vi "CoolLED_Control_v1.0.vi"(8 "error in":errorcluster) -> (0 "error out":errorcluster)   [LabVIEW 2025]
uses:
  SubVIs/States.ctl
  <vilib>/Instr/_visa.llb/VISA Configure Serial Port (Instr).vi
panel:
  in  "Tab Control":enum32{"Commands", "Expert"}(tab)
  in  "Presets":enum16{"DAPI", "GFP", "RFP", "None", "Multiple"}(ring)=enum."None"
  in  "Store":bool
  in  "Cluster":T1 {"Green-Red" step=1 scale=0.0..100.0; "Blue" step=1 scale=0.0..100.0; "Violet" step=1 scale=0.0..100.0}
  in  "VISA resource name":refnum<visa-resource-name>="COM5"
  out "Current command":string="CSSAXF000BXF000CXF000\r\n"
  in  "Stop":bool
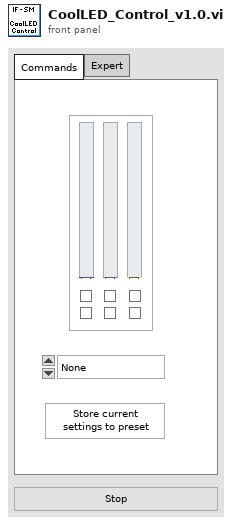
[diagram p1: front panel]
types:
  T1 = cluster{"Violet":u8, "Blue":u8, "Green-Red":u8, "A(S)Selected/(N)Unselected":bool, "B(S)Selected/(N)Unselected":bool, "C(S)Selected/(N)Unselected":bool, "A(N)ON/(F)OFF":bool, "(N)ON/(F)OFF":bool, "C(N)ON/(F)OFF":bool}
  T2 = typedef "States.ctl" = enum16{"Initialize", "Wait for Event", "Close", "Store", "Send", "Create_command", "Presets"}
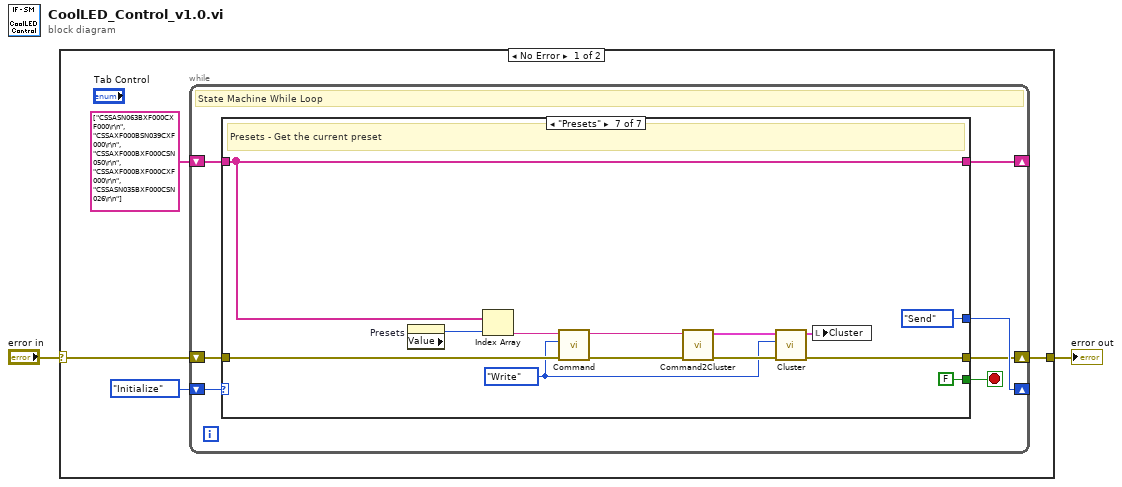
[diagram p0: block diagram]
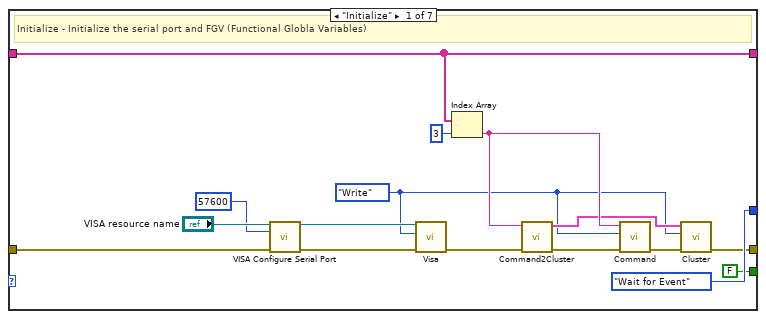
[diagram p2: hidden frame]
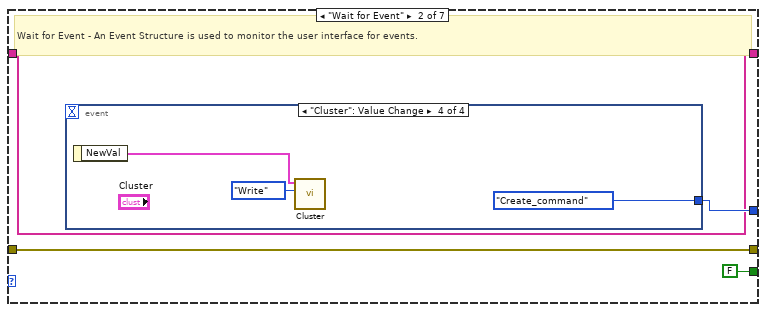
[diagram p3: hidden frame]
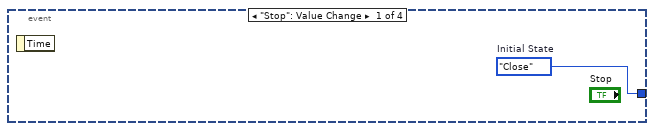
[diagram p4: hidden frame]
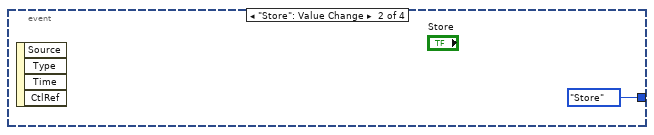
[diagram p5: hidden frame]
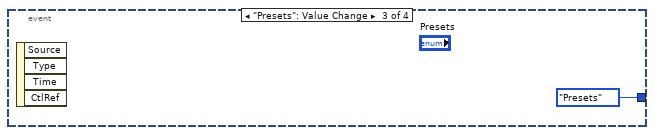
[diagram p6: hidden frame]
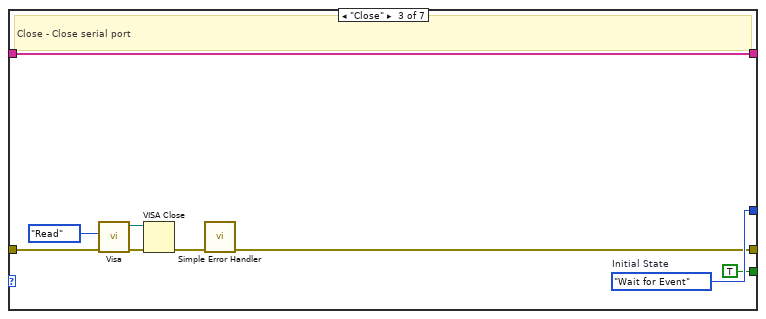
[diagram p7: hidden frame]
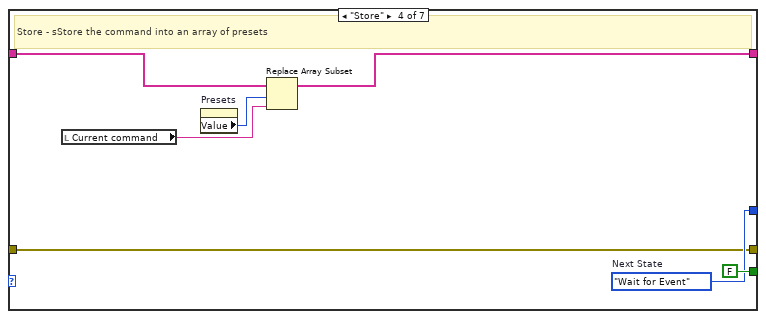
[diagram p8: hidden frame]
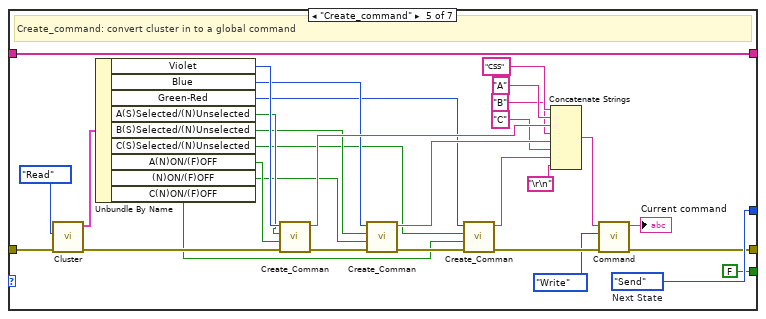
[diagram p9: hidden frame]
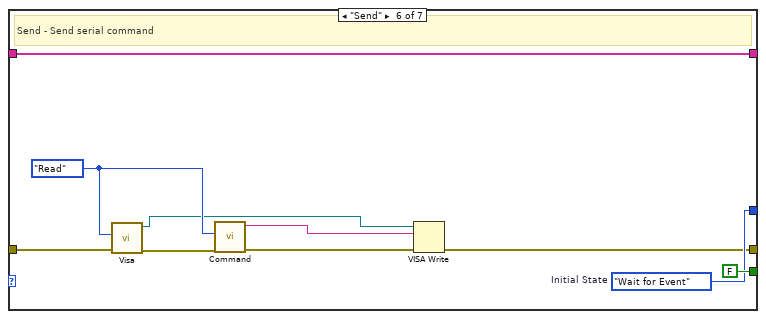
[diagram p10: hidden frame]
diagram:
  n1 = case shown="No Error" "error in" {
    selector: "error in" -> [w5 w110]
    tunnel: [w4 w110] -> w1
    frame No Error {
      n2 = while {
        shift-right: [w13] -> _
        shift-left: States."Initialize" ("Initial State") -> [w11]
        shift-right: [w9] -> w4
        shift-left: w5 -> [w10]
        shift-right: [w7] -> _
        shift-left: string[] ["CSSASN063BXF000CXF000\r\n", "CSSAXF000BSN039CXF000\r\n", "CSSAXF000BXF000CSN050\r\n", "CSSAXF000BXF000CXF000\r\n", "CSSASN035BXF000CSN026\r\n"] ("output array") -> [w8]
        stop <- w12 stop-if-true
        # "State Machine While Loop"
        n3 = case "State Machine Case Structure" shown="\"Presets\"" w11 {
          tunnel: [States."Wait for Event" ("Initial State") w33 w48 w54 w86 w95 States."Send" ("Initial State")] -> w13
          tunnel: [FALSE ("Stop the Loop") FALSE ("Stop the Loop") TRUE ("Stop the Loop") FALSE ("Stop the Loop") FALSE ("Stop the Loop") FALSE ("Stop the Loop") FALSE ("Stop the Loop")] -> w12
          tunnel: w10 -> [w26 w31 w43 w53 w68 w90 w106]
          tunnel: [w16 w31 w45 w53 w70 w92 w99] -> w9
          tunnel: w8 -> [w21 w30 w40 w52 w75 w94 w104]
          tunnel: [w21 w30 w40 w49 w75 w94 w104] -> w7
          frame "Initialize" {
            w14 = enum16{"Write", "Read"}."Write" ("Action")
            # "Initialize - Initialize the serial port and FGV (Functional Globla Variables)"
            n4 = call-poly "VISA Configure Serial Port"("VISA resource name"="VISA resource name", "baud rate (9600)"=u32 57600, "error in (no error)"=w26) -> ("VISA resource name out"=w24:refnum<visa-resource-name>, "error out"=w23:errorcluster)  [unwired: 6 in, 5 out]
            n5 = call "Visa.vi"("error in"=w23, "Action"=w14, "VISA resource name"=w24) -> ("error out"=w22:errorcluster)  [unwired: 7 in, 1 out]
            n6 = Index Array(array=w21, index=3) -> (element=w19:string)
            n7 = call "Command2Cluster.vi"("error in"=w22, "Current command"=w19) -> ("error out"=w18:errorcluster, "Cluster"=w15:T1)  [unwired: 8 in]
            n8 = call "Command.vi"("error in"=w18, "Action"=w14, "Command"=w19) -> ("error out"=w17:errorcluster)  [unwired: 7 in, 1 out]
            n9 = call "Cluster.vi"("error in"=w17, "Action"=w14, "Cluster"=w15) -> ("error out"=w16:errorcluster)  [unwired: 7 in, 1 out]
          }
          frame "Wait for Event" {
            # "Wait for Event - An Event Structure is used to monitor the user interface for events."
            n10 = event shown="[3] \"Cluster\": Value Change" {
              selector: _ -> [_ _ _ _]
              dyn-events: _ -> [_ _ _ _]
              timeout: _ -> [_ _ _ _]
              tunnel: [w34 States."Store" ("Initial State") States."Presets" ("Initial State") States."Create_command" ("Initial State")] -> w33
              event "Stop": Value Change {
                w34 = States."Close"  # Initial State
                n11 = event-data() -> ()  [unwired: 1 in, 1 out]
              }
              event "Store": Value Change {
                n12 = event-data() -> ()  [unwired: 1 in, 4 out]
              }
              event "Presets": Value Change {
                n13 = event-data() -> ()  [unwired: 1 in, 4 out]
              }
              event "Cluster": Value Change {
                n14 = event-data() -> ("NewVal"=w38:T1)  [unwired: 1 in]
                n15 = call "Cluster.vi"("Action"=enum16{"Write", "Read"}."Write", "Cluster"=w38) -> ()  [unwired: 8 in, 2 out]
              }
            }
          }
          frame "Close" {
            w48 = States."Wait for Event"  # Initial State
            # "Close - Close serial port"
            n16 = call "Visa.vi"("error in"=w43, "Action"=enum16{"Write", "Read"}."Read") -> ("error out"=w44:errorcluster, "VISA resource name"=w41:refnum<visa-resource-name>)  [unwired: 8 in]
            n17 = VISA Close(VISA resource name=w41, error in (no error)=w44) -> (error out=w46:errorcluster)
            n18 = call <vilib>:"Simple Error Handler.vi"("error in (no error)"=w46) -> ("error out"=w45:errorcluster)  [unwired: 1 in, 7 out]
          }
          frame "Store" {
            w54 = States."Wait for Event"  # Next State
            # "Store - sStore the command into an array of presets"
            n19 = local read "Current command"() -> (w50:string)
            n20 = property on="Presets" class="Enum (strict)"() -> ("Value"=w51:enum16{"DAPI", "GFP", "RFP", "None", "Multiple"})  [unwired: 2 in, 2 out]
            n21 = Replace Array Subset(array=w52, new element=w50, index=w51) -> (w49:string[])
          }
          frame "Create_command" {
            w86 = States."Send"  # Next State
            # "Create_command: convert cluster in to a global command"
            n22 = call "Cluster.vi"("error in"=w68, "Action"=enum16{"Write", "Read"}."Read") -> ("error out"=w67:errorcluster, "Cluster"=w65:T1)  [unwired: 8 in]
            n23 = Unbundle By Name(w65) -> ("Violet"=w64:u8, "Blue"=w63:u8, "Green-Red"=w62:u8, "A(S)Selected/(N)Unselected"=w61:bool, "B(S)Selected/(N)Unselected"=w60:bool, "C(S)Selected/(N)Unselected"=w59:bool, "A(N)ON/(F)OFF"=w58:bool, "(N)ON/(F)OFF"=w57:bool, "C(N)ON/(F)OFF"=w56:bool)
            n24 = call "Create_Comman.vi"("error in"=w67, "On/OFF"=w58, "Select"=w61, "Intensity"=w64) -> ("error out"=w84:errorcluster, "Command"=w80:string)  [unwired: 6 in]
            n25 = call "Create_Comman.vi"("error in"=w84, "On/OFF"=w57, "Select"=w60, "Intensity"=w63) -> ("error out"=w83:errorcluster, "Command"=w78:string)  [unwired: 6 in]
            n26 = call "Create_Comman.vi"("error in"=w83, "On/OFF"=w56, "Select"=w59, "Intensity"=w62) -> ("error out"=w73:errorcluster, "Command"=w76:string)  [unwired: 6 in]
            n27 = Concatenate Strings("CSS" ("string"), "A" ("string"), w80, "B" ("string"), w78, "C" ("string"), w76, "\r\n") -> (w72:string)
            n28 = call "Command.vi"("error in"=w73, "Action"=enum16{"Write", "Read"}."Write", "Command"=w72) -> ("error out"=w70:errorcluster, "Command"=→"Current command":string)  [unwired: 7 in]
          }
          frame "Send" {
            w88 = enum16{"Write", "Read"}."Read" ("Action")
            w95 = States."Wait for Event"  # Initial State
            # "Send - Send serial command"
            n29 = call "Visa.vi"("error in"=w90, "Action"=w88) -> ("error out"=w89:errorcluster, "VISA resource name"=w87:refnum<visa-resource-name>)  [unwired: 8 in]
            n30 = call "Command.vi"("error in"=w89, "Action"=w88) -> ("error out"=w93:errorcluster, "Command"=w91:string)  [unwired: 8 in]
            n31 = VISA Write(VISA resource name=w87, write buffer=w91, error in (no error)=w93) -> (error out=w92:errorcluster)  [unwired: 2 out]
          }
          frame "Presets" {
            w98 = enum16{"Write", "Read"}."Write" ("Action")
            # "Presets - Get the current preset"
            n32 = property on="Presets" class="Enum (strict)"() -> ("Value"=w107:enum16{"DAPI", "GFP", "RFP", "None", "Multiple"})  [unwired: 2 in, 2 out]
            n33 = Index Array(array=w104, index=w107) -> (element=w105:string)
            n34 = call "Command.vi"("error in"=w106, "Action"=w98, "Command"=w105) -> ("error out"=w100:errorcluster, "Command"=w103:string)  [unwired: 7 in]
            n35 = call "Command2Cluster.vi"("error in"=w100, "Current command"=w103) -> ("error out"=w101:errorcluster, "Cluster"=w102:T1)  [unwired: 8 in]
            n36 = call "Cluster.vi"("error in"=w101, "Action"=w98, "Cluster"=w102) -> ("error out"=w99:errorcluster, "Cluster"=w97:T1)  [unwired: 7 in]
            n37 = local write "Cluster"(w97) -> ()
          }
        }
      }
    }
    frame Error {
    }
  }
  "error out" <- w1
